vi "GetValue.vi"(8 "error in (no error)":errorcluster, 11 "TestClass in":refnum<class "TestClass.lvclass">) -> (0 "error out":errorcluster, 2 "Value":i32, 3 "TestClass out":refnum<class "TestClass.lvclass">)   [LabVIEW 2020, in "TestClass.lvclass"]
doc: "Provides a Get method for the TestClass"
uses:
  TestClass.lvclass
  TestClass.lvclass/TestClass.ctl
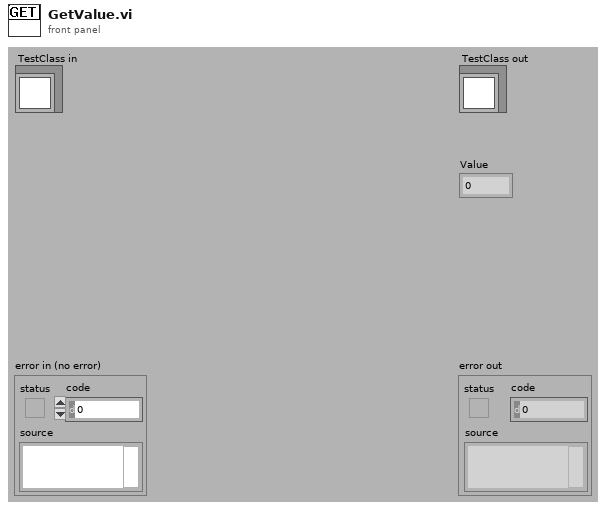
[diagram p1: front panel]
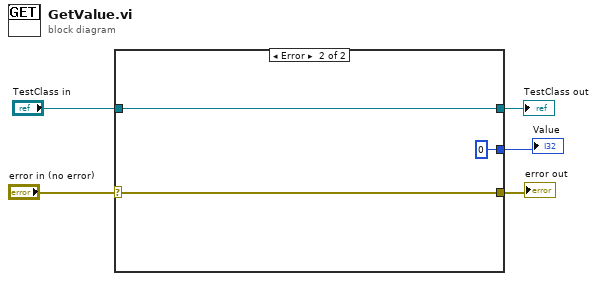
[diagram p0: block diagram]
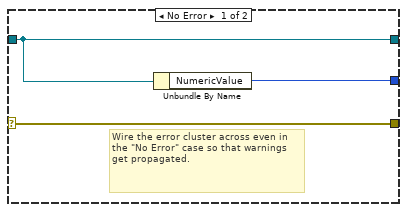
[diagram p2: hidden frame]
diagram:
  n1 = case shown="Error" "error in (no error)" {
    selector: "error in (no error)" -> [w8 w11]
    tunnel: [w8 w11] -> w4
    tunnel: [w7 w10] -> w2
    tunnel: "TestClass in" -> [w7 w10]
    tunnel: [w6 0 ("NumericValue")] -> w1
    frame No Error {
      # "Wire the error cluster across even in the \"No Error\" case so that warnings get propagated."
      n2 = Unbundle By Name(w7) -> ("NumericValue"=w6:i32)
    }
    frame Error {
    }
  }
  "error out" <- w4
  "TestClass out" <- w2
  "Value" <- w1
